vi "CLD 2  Elapsed Time Express FGV Solution.vi"(7 "Timer-Modus":T1, 8 "Fehler (Eingang, kein Fehler)":errorcluster, 9 "Autom. zurücksetzen (F)":bool, 11 "Zielzeit (s)":dbl) -> (0 "Fehler (Ausgang)":errorcluster, 2 "Verstrichene Zeit (s)":dbl format="%#.3g", 3 "Zeit ist verstrichen":bool)   [LabVIEW 2014]
doc: "CLD-Übung 2\n\nDieses SubVI ist eine FGV, die als Wrapper für das Express-VI dient. \n\nPer Voreinstellung wird durch das Zurücksetzen der FGV der Eingang \"Autom. zurücksetzen\" (und das Schieberegister) auf FALSE gesetzt. Das trifft nur zu, wenn der Case \"Autom. Zurücksetzen festlegen\" verwendet wird. \"Autom. zurücksetzen\" muss als separater Aufruf der FGV festgelegt werden.\n\nDamit diese Funktionsweise beobachtet werden kann, muss sich das VI im Speicher befinden. Zum Testen der FGV wurde ein Aufrufer-VI erstellt. Dies ist ein einfaches aufrufendes VI mit einer Schleife (ähnlich der Lösung in CLD-Übung 1)."
uses:
  CLD 2 Time Mode.ctl
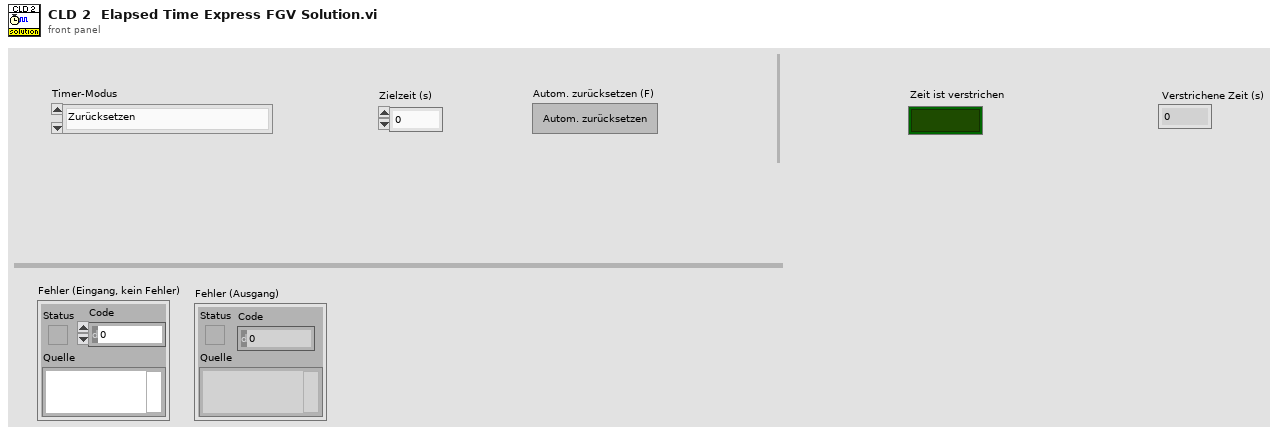
[diagram p1: front panel]
types:
  T1 = typedef "CLD 2 Time Mode.ctl" = enum16{"Zurücksetzen", "Status abfragen", "Autom. Zurücksetzen festlegen"}
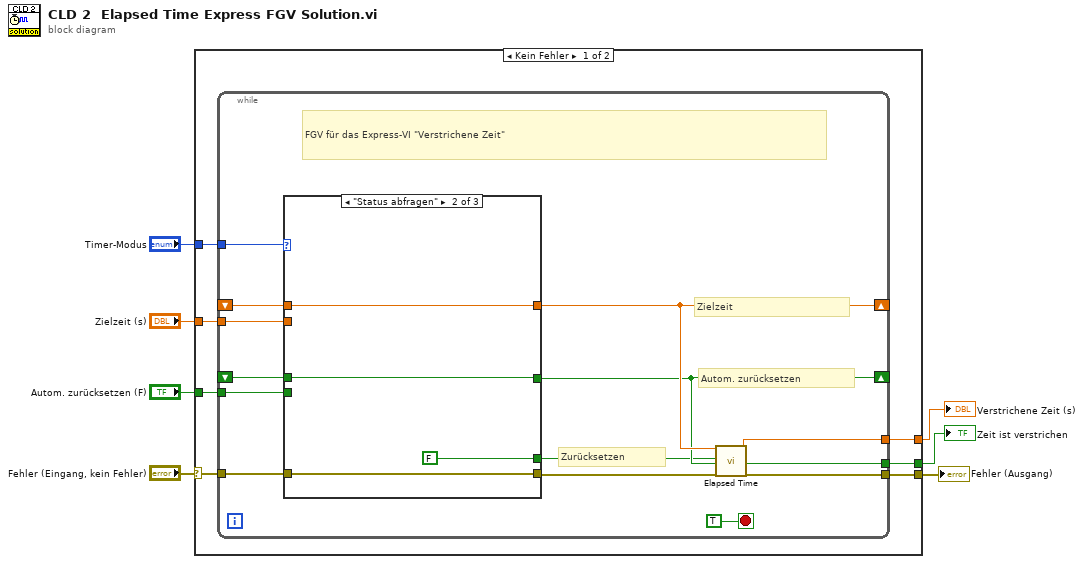
[diagram p0: block diagram]
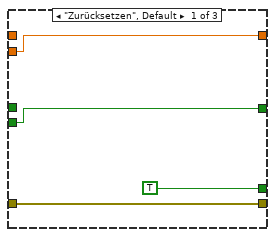
[diagram p2: hidden frame]
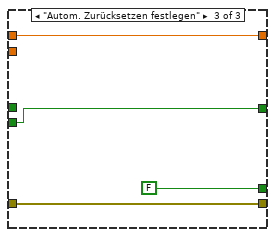
[diagram p3: hidden frame]
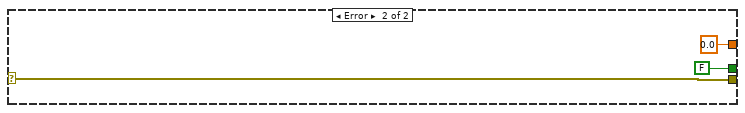
[diagram p4: hidden frame]
diagram:
  n1 = case shown="Kein Fehler" "Fehler (Eingang, kein Fehler)" {
    selector: "Fehler (Eingang, kein Fehler)" -> [w10 w43]
    tunnel: "Zielzeit (s)" -> [w14 _]
    tunnel: "Autom. zurücksetzen (F)" -> [w13 _]
    tunnel: "Timer-Modus" -> [w12 _]
    tunnel: [w11 w43] -> w4
    tunnel: [w9 0.0 ("Verstrichene Zeit (s)")] -> w2
    tunnel: [w8 FALSE ("Zeit ist verstrichen")] -> w1
    frame No Error {
      n2 = while {
        tunnel: w12 -> [w28]
        shift-right: [w25] -> _
        shift-left: _ -> [w27]
        shift-right: [w22] -> _
        shift-left: _ -> [w24]
        tunnel: w14 -> [w26]
        tunnel: w13 -> [w23]
        tunnel: w10 -> [w19]
        tunnel: [w17] -> w11
        tunnel: [w16] -> w9
        tunnel: [w15] -> w8
        stop <- TRUE stop-if-true
        # "Zielzeit"
        # "Autom. zurücksetzen"
        # "Zurücksetzen"
        # "FGV für das Express-VI \"Verstrichene Zeit\""
        n3 = case shown="\"Status abfragen\"" w28 {
          tunnel: w27 -> [_ w36 w40]
          tunnel: [w32 w36 w40] -> w25
          tunnel: w26 -> [w32 _ _]
          tunnel: w24 -> [_ w34 _]
          tunnel: [w31 w34 w39] -> w22
          tunnel: w23 -> [w31 _ w39]
          tunnel: [TRUE FALSE FALSE] -> w21
          tunnel: w19 -> [w29 w33 w37]
          tunnel: [w29 w33 w37] -> w18
          frame "Zurücksetzen", Default {
          }
          frame "Status abfragen" {
          }
          frame "Autom. Zurücksetzen festlegen" {
          }
        }
        n4 = call "Elapsed Time"("Time Target (s)"=w25, "Reset"=w21, "Auto Reset"=w22, "error in (no error)"=w18) -> ("Elapsed Time (s)"=w16:dbl, "Time has Elapsed"=w15:bool, "error out"=w17:errorcluster)  [unwired: 8 in, 5 out]
      }
    }
    frame Error {
    }
  }
  "Fehler (Ausgang)" <- w4
  "Zeit ist verstrichen" <- w1
  "Verstrichene Zeit (s)" <- w2
